vi "PRBS.vi"(7 "Frequency Divider":u32=1 min=1 step=1, 8 "Amplitude":dbl min=0.0, 9 "Periods":u32=1 min=1 step=1, 10 "Reference":u16(ring) items=["Change X", "Change Y"], 11 "Order":u32=1 min=1 step=1) -> (3 "appended array":dbl[][](array[numeric]))   [LabVIEW 2021, in "System.lvclass"]
uses:
  System.lvclass
panel:
  out "size(s)":i32
  out "x-y":i32[](array[numeric])
  out "PRBS":i32[](array[numeric])
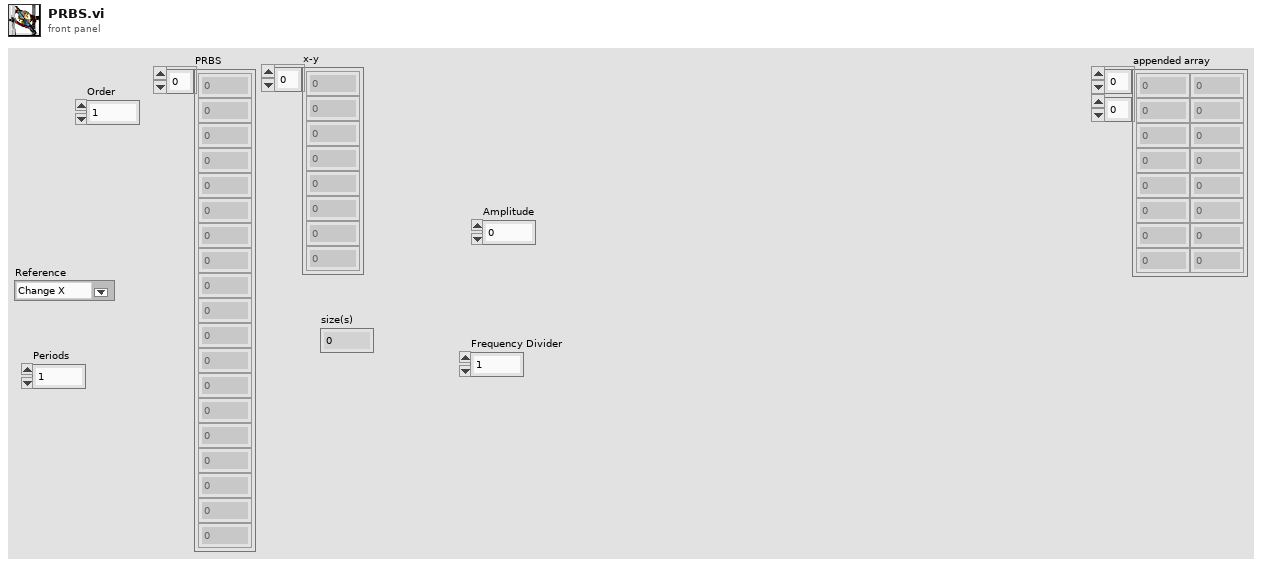
[diagram p1: front panel]
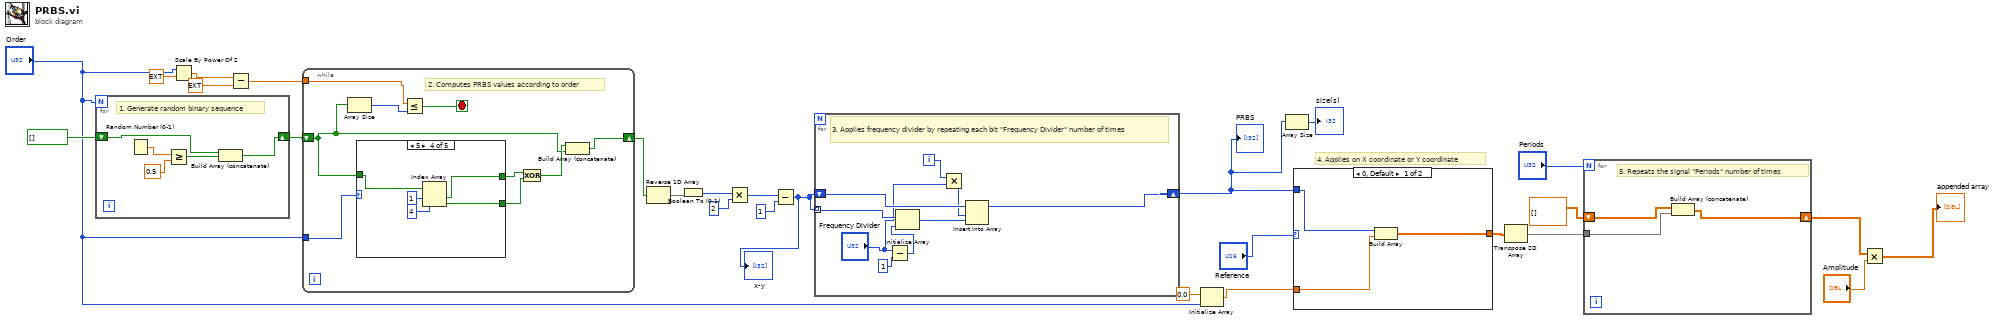
[diagram p0: block diagram]
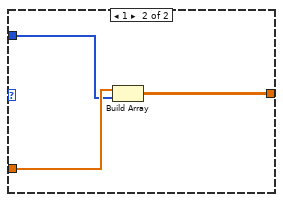
[diagram p2: hidden frame]
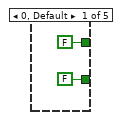
[diagram p3: hidden frame]
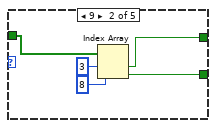
[diagram p4: hidden frame]
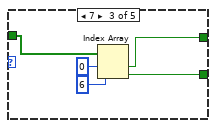
[diagram p5: hidden frame]
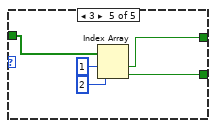
[diagram p6: hidden frame]
diagram:
  # "4. Applies on X coordinate or Y coordinate"
  n1 = for {
    N: "Order" -> [_]
    shift-right: [w27] -> w25
    shift-left: bool[] [] -> [w28]
    # "1. Generate random binary sequence"
    n2 = Random Number (0-1)() -> (number: 0 to 1=w31:dbl)
    n3 = Greater Or Equal?(x=w31, y=0.5) -> (x >= y?=w29:bool)
    n4 = Build Array (concatenate)(w28, w29) -> (w27:bool[])
  }
  n5 = Scale By Power Of 2(n="Order", x=ext 1.0) -> (x*2^n=w18:ext)
  n6 = Subtract(x=w18, y=ext 2.0) -> (x-y=w16:ext)
  n7 = while {
    tunnel: "Order" -> [w40]
    shift-right: [w37] -> w26
    shift-left: w25 -> [w35]
    tunnel: w16 -> [w32]
    stop <- w33 stop-if-true
    # "2. Computes PRBS values according to order"
    n8 = Array Size(array=w35) -> (size(s)=w34:i32)
    n9 = case shown="5" w40 {
      tunnel: w35 -> [_ w47 w52 w57 w62]
      tunnel: [FALSE ("element") w46 w51 w56 w61] -> w39
      tunnel: [FALSE ("element") w45 w50 w55 w60] -> w38
      frame 0, Default {
      }
      frame 9 {
        n10 = Index Array(array=w47, index #1=3 ("index"), index #2=8 ("index")) -> (element #1=w46:bool, element #2=w45:bool)
      }
      frame 7 {
        n11 = Index Array(array=w52, index #1=0 ("index"), index #2=6 ("index")) -> (element #1=w51:bool, element #2=w50:bool)
      }
      frame 5 {
        n12 = Index Array(array=w57, index #1=1 ("index"), index #2=4 ("index")) -> (element #1=w56:bool, element #2=w55:bool)
      }
      frame 3 {
        n13 = Index Array(array=w62, index #1=1 ("index"), index #2=2 ("index")) -> (element #1=w61:bool, element #2=w60:bool)
      }
    }
    n14 = Less Or Equal?(x=w32, y=w34) -> (x <= y?=w33:bool)
    n15 = Compound Arithmetic op=XOR(w39, w38) -> (w36:bool)
    n16 = Build Array (concatenate)(w36, w35) -> (w37:bool[])
  }
  n17 = Reverse 1D Array(array=w26) -> (reversed array=w24:bool[])
  n18 = Boolean To (0,1)(Boolean=w24) -> (0, 1=w23:i16[])
  n19 = Multiply(x=w23, y=2) -> (x*y=w22:i32[])
  n20 = Subtract(x=w22, y=1) -> (x-y=w1:i32[])
  "x-y" <- w1
  n21 = for {
    shift-right: [w67] -> w3
    shift-left: w1 -> [w68]
    tunnel: w1 -> [w71] mode=indexing
    i -> [w64]
    # "3. Applies frequency divider by repeating each bit \"Frequency Divider\" number of times"
    n22 = Subtract(x="Frequency Divider", y=u32 1) -> (x-y=w70:u32)
    n23 = Initialize Array(w71, w70) -> (w66:i32[])
    n24 = Multiply(x=w64, y="Frequency Divider") -> (x*y=w63:u32)
    n25 = Insert Into Array(array=w68, index=w63, new element=w66) -> (w67:i32[])
  }
  "PRBS" <- w3
  n26 = Initialize Array(0.0 ("element"), "Order") -> (w11:dbl[])
  n27 = Array Size(array=w3) -> (size(s)=→"size(s)":i32)
  n28 = case shown="0, Default" "Reference" {
    tunnel: w11 -> [w73 w77]
    tunnel: w3 -> [w74 w76]
    tunnel: [w72 w75] -> w10
    frame 0, Default {
      n29 = Build Array(w74, w73) -> (w72:dbl[][])
    }
    frame 1 {
      n30 = Build Array(w77, w76) -> (w75:dbl[][])
    }
  }
  n31 = Transpose 2D Array(2D array=w10) -> (transposed array=w8:dbl[][])
  n32 = for {
    N: "Periods" -> [_]
    tunnel: w8 -> [w79]
    shift-right: [w78] -> w5
    shift-left: dbl[][] [] -> [w80]
    # "5. Repeats the signal \"Periods\" number of times"
    n33 = Build Array (concatenate)(w80, w79) -> (w78:dbl[][])
  }
  n34 = Multiply(x=w5, y="Amplitude") -> (x*y=→"appended array":dbl[][])
